vi "myRIO v1.2 Open Throughput AudioIn (N Samples).vi"(7 "Allow multiple opens?":bool, 8 "error in (no error)":errorcluster, 10 "Channel Names":string[](array[string]), 11 "Resource name":T5 caption="RIO Device") -> (0 "error out":errorcluster, 1 "AudioIn (N Samples) Scale Constants List":T1, 2 "AudioIn (N Samples) Channel List":T6, 3 "myRIO Ref Out":T3)   [LabVIEW 2021]
uses:
  <vilib>/myRIO/Common/Instrument Driver Framework/myRIO v1.0/AudioIn Block/typedefs/AudioIn Block Channels List.ctl
  <vilib>/myRIO/Common/Instrument Driver Framework/myRIO v1.0/AudioIn Block/typedefs/AudioIn Block Channels Enum.ctl
  <vilib>/userDefined/High Color/nirio_resource_hc.ctl
  <vilib>/myRIO/Common/Instrument Driver Framework/Utilities/typedefs/myRIO v1.0 Reference.ctl
  <vilib>/myRIO/Common/Instrument Driver Framework/Utilities/typedefs/Generic FPGA Reference.ctl
  <vilib>/myRIO/Common/Instrument Driver Framework/Utilities/typedefs/Analog Scaling Constants List.ctl
  <vilib>/myRIO/Common/Instrument Driver Framework/Utilities/typedefs/Analog Scaling Constants.ctl
  <vilib>/myRIO/Common/Instrument Driver Framework/myRIO v1.0/AudioIn Block/typedefs/myRIO v1.2 AudioIn Block Channels Enum.ctl
  <vilib>/Utility/VariantDataType/GetNumericInfo.vi
  <vilib>/Utility/error.llb/Error Cluster From Error Code.vi
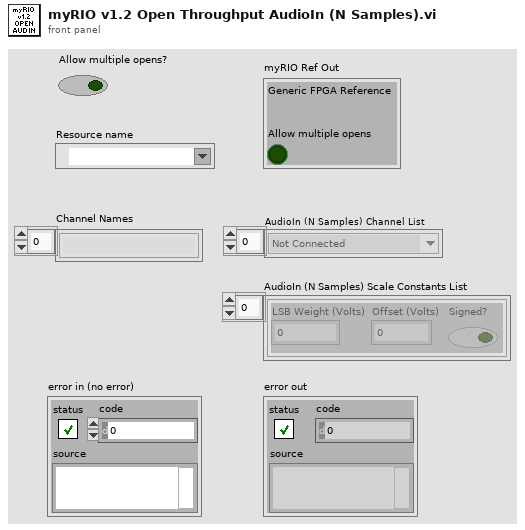
[diagram p1: front panel]
types:
  T1 = typedef "Analog Scaling Constants List.ctl" = T2[]
  T2 = typedef "Analog Scaling Constants.ctl" = cluster{"LSB Weight (Volts)":dbl, "Offset (Volts)":dbl, "Signed?":bool}
  T3 = typedef "myRIO v1.0 Reference.ctl" = cluster{"Generic FPGA Reference":T4, "Allow multiple opens":bool}
  T4 = typedef "Generic FPGA Reference.ctl" = refnum<k20>
  T5 = typedef "nirio_resource_hc.ctl" = tag
  T6 = typedef "AudioIn Block Channels List.ctl" = T7[]
  T7 = typedef "AudioIn Block Channels Enum.ctl" = enum16{"Not Connected", "AudioIn/Left (N Samples)", "AudioIn/Right (N Samples)"}
  T8 = typedef "myRIO v1.2 AudioIn Block Channels Enum.ctl" = enum16{"Not Connected"}
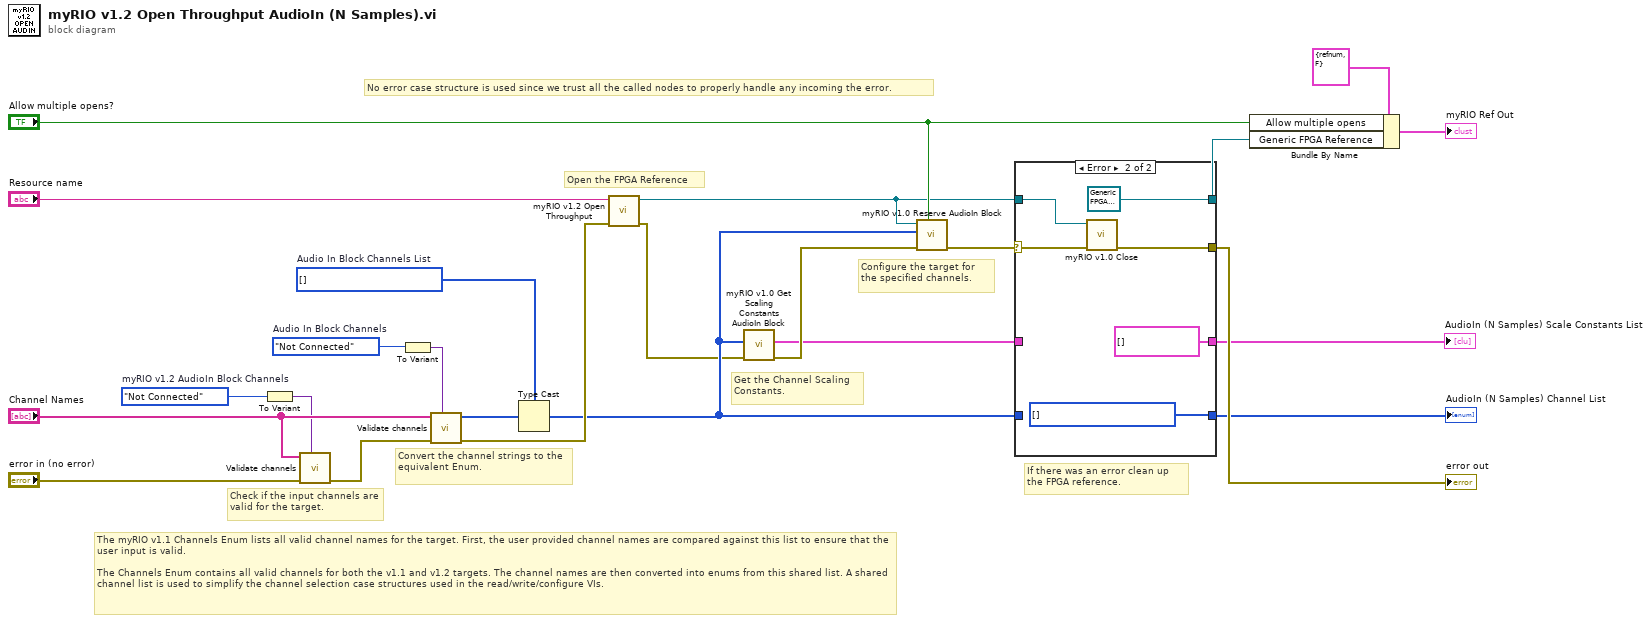
[diagram p0: block diagram]
diagram:
  w7 = T6 [] items=["Not Connected", "AudioIn/Left (N Samples)", "AudioIn/Right (N Samples)"]  # Audio In Block Channels List
  w8 = AudioIn_Block_Channels_Enum."Not Connected"  # Audio In Block Channels
  w9 = myRIO_v1.2_AudioIn_Block_Channels_Enum."Not Connected"  # myRIO v1.2 AudioIn Block Channels
  # "Get the Channel Scaling Constants."
  # "The myRIO v1.1 Channels Enum lists all valid channel names for the target. First, the user provided channel names are compared against this list to ensure that the user input is valid.\n\nThe Channels Enum contains all valid channels for both the v1.1 and v1.2 targets. The channel names are then converted into enums from this shared list. A shared channel list is used to simplify the channel selection case structures used in the read/write/configure VIs."
  # "If there was an error clean up the FPGA reference."
  # "Configure the target for the specified channels."
  # "Open the FPGA Reference"
  # "No error case structure is used since we trust all the called nodes to properly handle any incoming the error."
  # "Convert the channel strings to the equivalent Enum."
  # "Check if the input channels are valid for the target."
  n1 = To Variant(anything=w9) -> (Variant=w12:variant)
  n2 = call <vilib>:"Validate channels.vi"("Channels Enum Variant"=w12, "error in (no error)"="error in (no error)", "Channel Names"="Channel Names") -> ("error out"=w23:errorcluster)  [unwired: 7 in, 1 out]
  n3 = To Variant(anything=w8) -> (Variant=w13:variant)
  n4 = call <vilib>:"Validate channels.vi"("Channels Enum Variant"=w13, "error in (no error)"=w23, "Channel Names"="Channel Names") -> ("error out"=w19:errorcluster, "Index Array"=w18:u16[])  [unwired: 7 in]
  n5 = Type Cast(type=w7, x=w18) -> (*(type *) &x=w6:T6)
  n6 = call <vilib>:"myRIO v1.2 Open Throughput.vi"("error in (no error)"=w19, "Resource name"="Resource name") -> ("error out"=w5:errorcluster, "myRIO FPGA Ref Out"=w1:T4)  [unwired: 8 in]
  n7 = call <vilib>:"myRIO v1.0 Get Scaling Constants AudioIn Block.vi"("error in (no error)"=w5, "AudioIn (N Samples) Channel List"=w6) -> ("error out"=w4:errorcluster, "Scale Constants Array"=w3:T1)  [unwired: 8 in]
  n8 = call <vilib>:"myRIO v1.0 Reserve AudioIn Block.vi"("Allow multiple opens?"="Allow multiple opens?", "error in (no error)"=w4, "AudioIn (N Samples) Channel List"=w6, "Generic FPGA Reference"=w1) -> ("error out"=w14:errorcluster)  [unwired: 7 in]
  n9 = case shown="Error" w14 {
    selector: w14 -> [w28 w34]
    tunnel: [w26 T4 refnum ("myRIO FPGA Ref Out")] -> w16
    tunnel: [w28 w33] -> w21
    tunnel: [w27 w30] -> w17
    tunnel: w6 -> [w27 _]
    tunnel: w1 -> [w26 w31]
    tunnel: w3 -> [w25 _]
    tunnel: [w25 T1 [] ("Scale Constants Array")] -> w2
    frame No Error {
    }
    frame Error {
      w30 = T6 [] items=["Not Connected", "AudioIn/Left (N Samples)", "AudioIn/Right (N Samples)"] ("Audio In Block Read Channels List")
      n10 = call <vilib>:"myRIO v1.0 Close.vi"("error in (no error)"=w34, "myRIO FPGA Ref In"=w31) -> ("error out"=w33:errorcluster)  [unwired: 9 in]
    }
  }
  "AudioIn (N Samples) Channel List" <- w17
  "error out" <- w21
  "AudioIn (N Samples) Scale Constants List" <- w2
  n11 = Bundle By Name(cluster=T3 {"Generic FPGA Reference"=refnum, "Allow multiple opens"=FALSE} ("myRIO Ref Out"), "Allow multiple opens"="Allow multiple opens?", "Generic FPGA Reference"=w16) -> (→"myRIO Ref Out":T3)
